vi "HW_ni_Search Devices in System.vi"(8 "error in":errorcluster caption="错误输入") -> (0 "error out":errorcluster caption="错误输出", 2 "DevicesInfo out":T1[](array[typedef]))   [LabVIEW 2016]
doc: "检测系统中的NI设备：\n包括机箱信息、模块信息、通道基本信息等。\n\n两种方式：\n1、配置文件中读取\n2、自动检测\n具体实现方式在配置文件中配置。"
uses:
  Ctrls/HardWare Basic Info _ Channel.ctl
  Ctrls/HardWare Basic Info _ Module.ctl
  Ctrls/HardWare Basic Info _ Chassis.ctl
  Ctrls/HardWare Basic Info _ Device.ctl
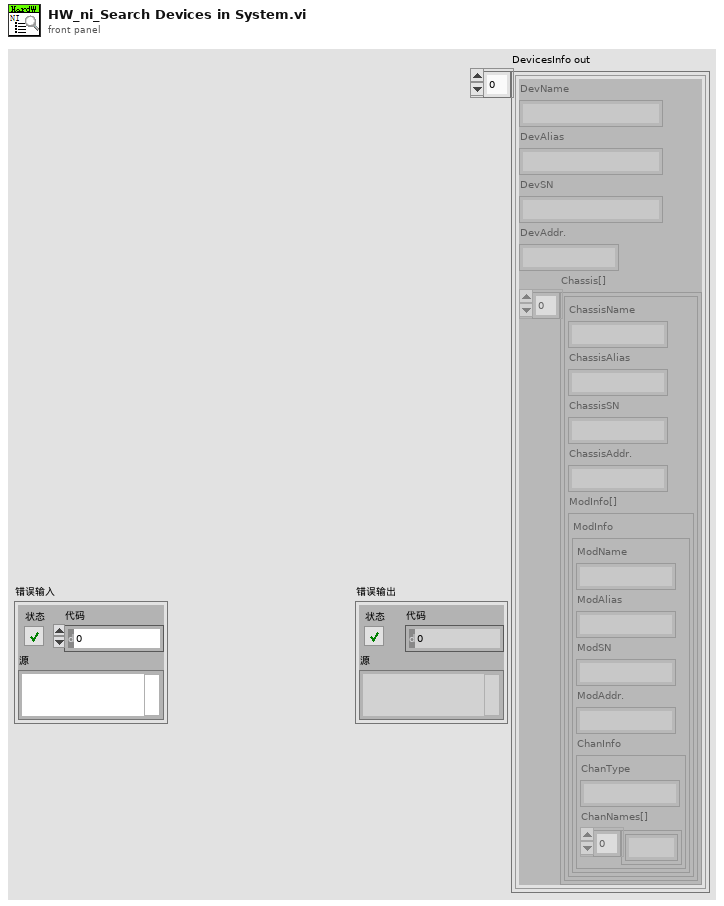
[diagram p1: front panel]
types:
  T1 = typedef "HardWare Basic Info _ Device.ctl" = cluster{"DevName":string, "DevAlias":string, "DevSN":string, "DevAddr.":string, "Chassis[]":T2[]}
  T2 = typedef "HardWare Basic Info _ Chassis.ctl" = cluster{"ChassisName":string, "ChassisAlias":string, "ChassisSN":string, "ChassisAddr.":string, "ModInfo[]":T3[]}
  T3 = typedef "HardWare Basic Info _ Module.ctl" = cluster{"ModName":string, "ModAlias":string, "ModSN":string, "ModAddr.":string, "ChanInfo":T4}
  T4 = typedef "HardWare Basic Info _ Channel.ctl" = cluster{"ChanType":string, "ChanNames[]":string[]}
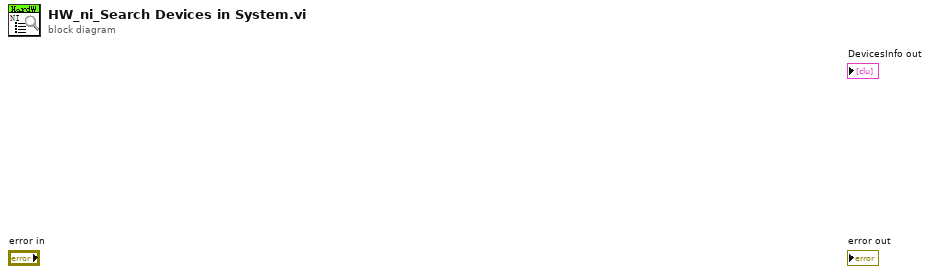
[diagram p0: block diagram]
diagram:
